vi "Required LV Version.vi"(8 "error in (no error)":errorcluster, 11 "Build Package Item in":refnum<class "VIPM Item.lvclass">) -> (0 "error out":errorcluster, 1 "64 Bit?":bool, 2 "LV Year":u32)   [LabVIEW 2019, in "VIPM.lvlib" / "VIPM Item.lvclass"]
uses:
  VIPM Item.lvclass
  VIPM Item.lvclass/VIPM Item.ctl
  <vilib>/xml/Load XML File.vi
  <vilib>/xml/Close Reference(Node).vi
  <vilib>/xml/NI_XML.lvlib
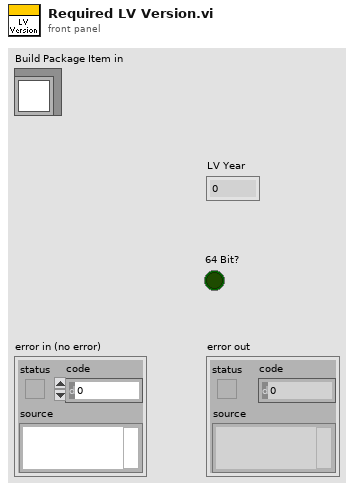
[diagram p1: front panel]
types:
  T1 = typedef "VIPM.lvlib/VIPM Item.lvclass/File Type.ctl" = enum16{"Unsupported", "VIPB", "VIPC"}
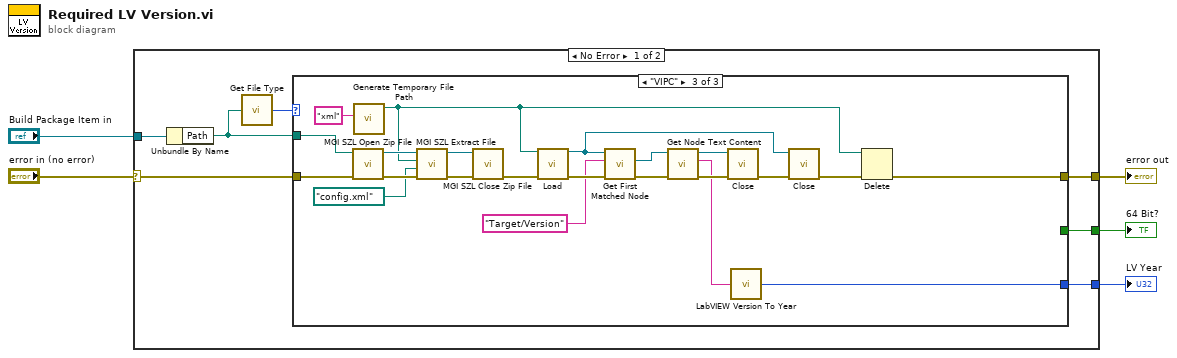
[diagram p0: block diagram]
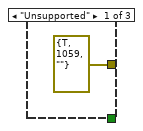
[diagram p2: hidden frame]
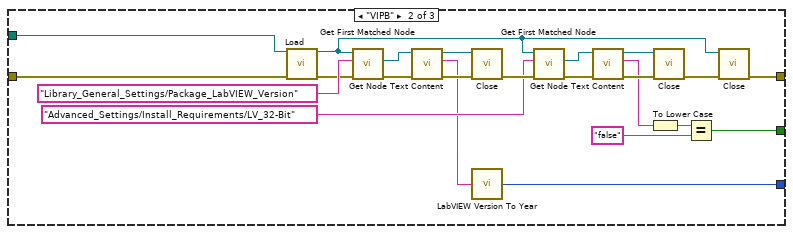
[diagram p3: hidden frame]
diagram:
  n1 = case shown="No Error" "error in (no error)" {
    selector: "error in (no error)" -> [w12 w59]
    tunnel: [w11 w59] -> w4
    tunnel: [w10 _] -> w3
    tunnel: "Build Package Item in" -> [w9 _]
    tunnel: [w8 _] -> w1
    frame No Error {
      n2 = Unbundle By Name(w9) -> ("Path"=w6:path)
      n3 = call "Get File Type.vi"("Path"=w6) -> ("File Type"=w7:T1)  [unwired: 1 in]
      n4 = case shown="\"VIPC\"" w7 {
        tunnel: w12 -> [_ w30 w58]
        tunnel: [errorcluster {"status"=TRUE, "code"=1059, "source"=""} ("error out") w29 w38] -> w11
        tunnel: [_ w14 w41] -> w10
        tunnel: w6 -> [_ w28 w57]
        tunnel: [_ w16 _] -> w8
        frame "Unsupported" {
        }
        frame "VIPB" {
          n5 = call-poly <vilib>:"Load.vi"("path to XML document"=w28, "error in (no error)"=w30) -> ("DOM document out"=w20:refnum<k20>, "error out"=w35:errorcluster)  [unwired: 11 in, 1 out]
          n6 = call <vilib>:"Get First Matched Node.vi"("error in (no error)"=w35, "XPath expression"="Library_General_Settings/Package_LabVIEW_Version", "node in"=w20) -> ("error out"=w33:errorcluster, "node result"=w34:refnum<k20>)  [unwired: 6 in, 1 out]
          n7 = call <vilib>:"Get Node Text Content.vi"("error in (no error)"=w33, "node in"=w34) -> ("error out"=w32:errorcluster, "node text"=w15:string, "node out"=w31:refnum<k20>)  [unwired: 7 in]
          n8 = call-poly <vilib>:"Close.vi"("error in (no error)"=w32, "node"=w31) -> ("error out"=w26:errorcluster)  [unwired: 7 in]
          n9 = call "LabVIEW Version To Year.vi"("LabVIEW Version"=w15) -> ("LabVIEW Year"=w14:u32)  [unwired: 1 in]
          n10 = call <vilib>:"Get First Matched Node.vi"("error in (no error)"=w26, "XPath expression"="Advanced_Settings/Install_Requirements/LV_32-Bit", "node in"=w20) -> ("error out"=w27:errorcluster, "node result"=w21:refnum<k20>)  [unwired: 6 in, 1 out]
          n11 = call <vilib>:"Get Node Text Content.vi"("error in (no error)"=w27, "node in"=w21) -> ("error out"=w25:errorcluster, "node text"=w19:string, "node out"=w24:refnum<k20>)  [unwired: 7 in]
          n12 = To Lower Case(string=w19) -> (all lower case string=w18:string)
          n13 = call-poly <vilib>:"Close.vi"("error in (no error)"=w25, "node"=w24) -> ("error out"=w23:errorcluster)  [unwired: 7 in]
          n14 = Equal?(x=w18, y="false") -> (x = y?=w16:bool)
          n15 = call-poly <vilib>:"Close.vi"("error in (no error)"=w23, "node"=w20) -> ("error out"=w29:errorcluster)  [unwired: 7 in]
        }
        frame "VIPC" {
          n16 = call <userlib>:"MGI SZL Open Zip File.vi"("Error In"=w58, "Existing Zip Path"=w57) -> ("Error Out"=w56:errorcluster, "Opened Zip File"=w55:refnum<k24>)  [unwired: 8 in]
          n17 = call <vilib>:"Generate Temporary File Path.vi"("Temporary File Extension (tmp)"="xml") -> ("Unique Temporary File Path"=w37:path)  [unwired: 9 in, 1 out]
          n18 = call <userlib>:"MGI SZL Extract File.vi"("Error In"=w56, "Entry Path In Zip"=path "config.xml", "Target Path"=w37, "Zip File"=w55) -> ("Error Out"=w52:errorcluster, "Zip File Out"=w51:refnum<k24>)  [unwired: 5 in, 1 out]
          n19 = call <userlib>:"MGI SZL Close Zip File.vi"("Error In"=w52, "Zip File"=w51) -> ("Error Out"=w50:errorcluster)  [unwired: 9 in]
          n20 = call-poly <vilib>:"Load.vi"("path to XML document"=w37, "error in (no error)"=w50) -> ("DOM document out"=w42:refnum<k20>, "error out"=w49:errorcluster)  [unwired: 11 in, 1 out]
          n21 = call <vilib>:"Get First Matched Node.vi"("error in (no error)"=w49, "XPath expression"="Target/Version", "node in"=w42) -> ("error out"=w47:errorcluster, "node result"=w45:refnum<k20>)  [unwired: 6 in, 1 out]
          n22 = call <vilib>:"Get Node Text Content.vi"("error in (no error)"=w47, "node in"=w45) -> ("error out"=w46:errorcluster, "node text"=w40:string, "node out"=w44:refnum<k20>)  [unwired: 7 in]
          n23 = call-poly <vilib>:"Close.vi"("error in (no error)"=w46, "node"=w44) -> ("error out"=w43:errorcluster)  [unwired: 7 in]
          n24 = call "LabVIEW Version To Year.vi"("LabVIEW Version"=w40) -> ("LabVIEW Year"=w41:u32)  [unwired: 1 in]
          n25 = call-poly <vilib>:"Close.vi"("error in (no error)"=w43, "node"=w42) -> ("error out"=w39:errorcluster)  [unwired: 7 in]
          n26 = Delete(path (use dialog)=w37, error in=w39) -> (error out=w38:errorcluster)  [unwired: 3 in, 2 out]
        }
      }
    }
    frame Error {
    }
  }
  "error out" <- w4
  "LV Year" <- w3
  "64 Bit?" <- w1
